vi "TB-Restore Defaults.vi"() -> (4 "Exposure parameters out":T1, 15 "error out":errorcluster)   [LabVIEW 2020]
uses:
  Typedefs/TB-Parameters.ctl
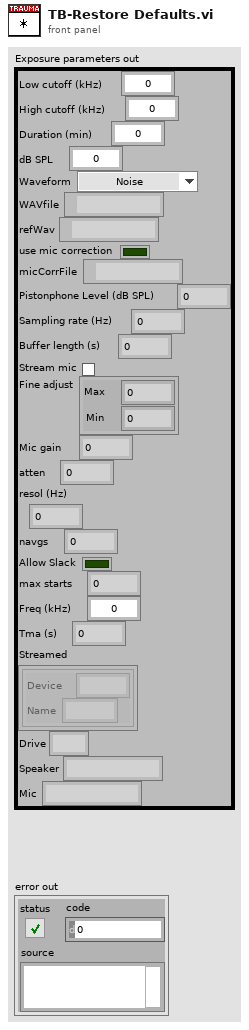
[diagram p1: front panel]
types:
  T1 = typedef "TB-Parameters.ctl" = cluster{"Low cutoff (kHz)":dbl, "High cutoff (kHz)":dbl, "Duration (min)":dbl, "dB SPL":dbl, "Waveform":enum16{"Noise", "File", "Tone"}, "WAVfile":path, "refWav":path, "use mic correction":bool, "micCorrFile":path, "Pistonphone Level (dB SPL)":dbl, "Sampling rate (Hz)":dbl, "Buffer length (s)":dbl, "Stream mic":bool, "Fine adjust":cluster{"Max":dbl, "Min":dbl}, "Mic gain":dbl, "atten":dbl, "resol (Hz)":dbl, "navgs":i32, "Allow Slack":bool, "max starts":i32, "Freq (kHz)":dbl, "Tma (s)":dbl, "Streamed":cluster{"Device":string, "Name":string}[], "Drive":string, "Speaker":string, "Mic":string}
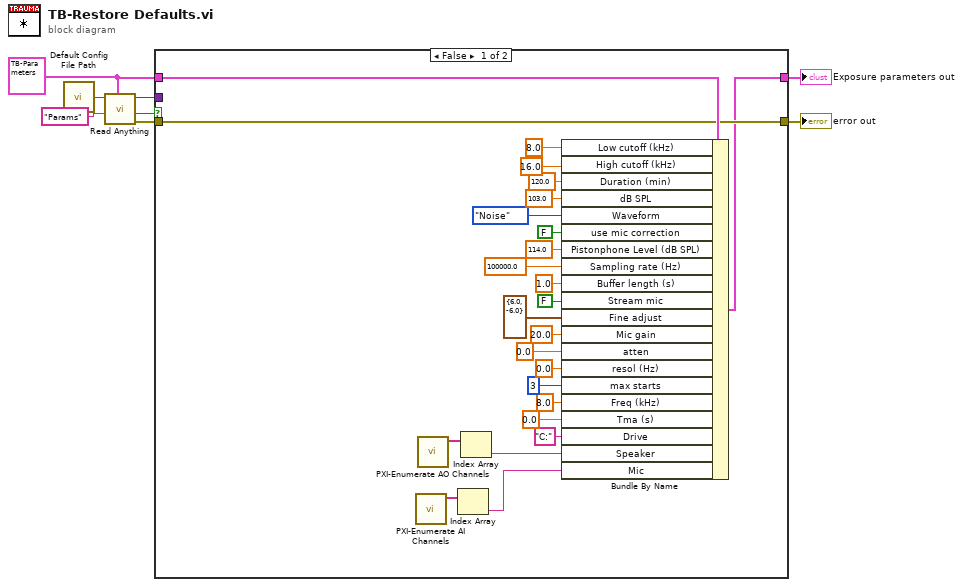
[diagram p0: block diagram]
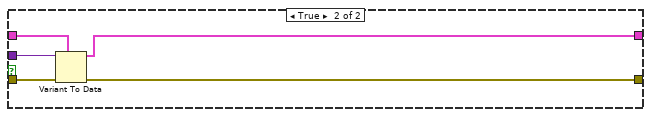
[diagram p2: hidden frame]
diagram:
  w2 = T1 {"Low cutoff (kHz)"=0.0, "High cutoff (kHz)"=0.0, "Duration (min)"=0.0, "dB SPL"=0.0, "Waveform"=enum."Noise", "WAVfile"=path "", "refWav"=path "", "use mic correction"=FALSE, "micCorrFile"=path "", "Pistonphone Level (dB SPL)"=0.0, "Sampling rate (Hz)"=0.0, "Buffer length (s)"=0.0, "Stream mic"=FALSE, "Fine adjust"={"Max"=0.0, "Min"=0.0}, "Mic gain"=0.0, "atten"=0.0, "resol (Hz)"=0.0, "navgs"=0, "Allow Slack"=FALSE, "max starts"=0, "Freq (kHz)"=0.0, "Tma (s)"=0.0, "Streamed"=[], "Drive"="", "Speaker"="", "Mic"=""} ("Exposure parameters out")
  n1 = call "Default Config File Path.vi"() -> ("Default config file name"=w5:path)
  n2 = call "Read Anything.vi"("Type of Anything"=w2, "Section Name (Name of \"Type of Anything\")"="Params" ("Section Name (Name of \"Type of Anything\")"), "Path (dialog)"=w5) -> ("Error Out"=w7:errorcluster, "Found?"=w8:bool, "Anything"=w6:variant)  [unwired: 6 in]
  n3 = case shown="False" w8 {
    tunnel: [w32 w38] -> w4
    tunnel: w6 -> [_ w37]
    tunnel: w7 -> [w32 w36]
    tunnel: [w31 w35] -> w1
    tunnel: w2 -> [w33 w34]
    frame False {
      n4 = call "PXI-Enumerate AI Channels.vi"() -> ("AI.PhysicalChans"=w11:tag[])  [unwired: 11 in]
      n5 = call "PXI-Enumerate AO Channels.vi"() -> ("AO.PhysicalChans"=w12:tag[])  [unwired: 11 in]
      n6 = Index Array(array=w11) -> (element=w9:tag)  [unwired: 1 in]
      n7 = Index Array(array=w12) -> (element=w10:tag)  [unwired: 1 in]
      n8 = Bundle By Name(cluster=w33, "Low cutoff (kHz)"=8.0, "High cutoff (kHz)"=16.0, "Duration (min)"=120.0, "dB SPL"=103.0, "Waveform"=enum16{"Noise", "File", "Tone"}."Noise", "use mic correction"=FALSE, "Pistonphone Level (dB SPL)"=114.0, "Sampling rate (Hz)"=100000.0, "Buffer length (s)"=1.0, "Stream mic"=FALSE, "Fine adjust"=cluster{"Max":dbl, "Min":dbl} {"Max"=6.0, "Min"=-6.0}, "Mic gain"=20.0, "atten"=0.0, "resol (Hz)"=0.0, "max starts"=3, "Freq (kHz)"=8.0, "Tma (s)"=0.0, "Drive"="C:", "Speaker"=w10, "Mic"=w9) -> (w31:T1)
    }
    frame True {
      n9 = Variant To Data(error in=w36, type=w34, Variant=w37) -> (data=w35:T1, error out=w38:errorcluster)
    }
  }
  "Exposure parameters out" <- w1
  "error out" <- w4
